vi "PID-control.vi"() -> ()   [LabVIEW 2012]
panel:
  out "Waveform Graph 2":dynamicdata(graph)
  in  "stop":bool
  out "Waveform Graph":dynamicdata(graph)
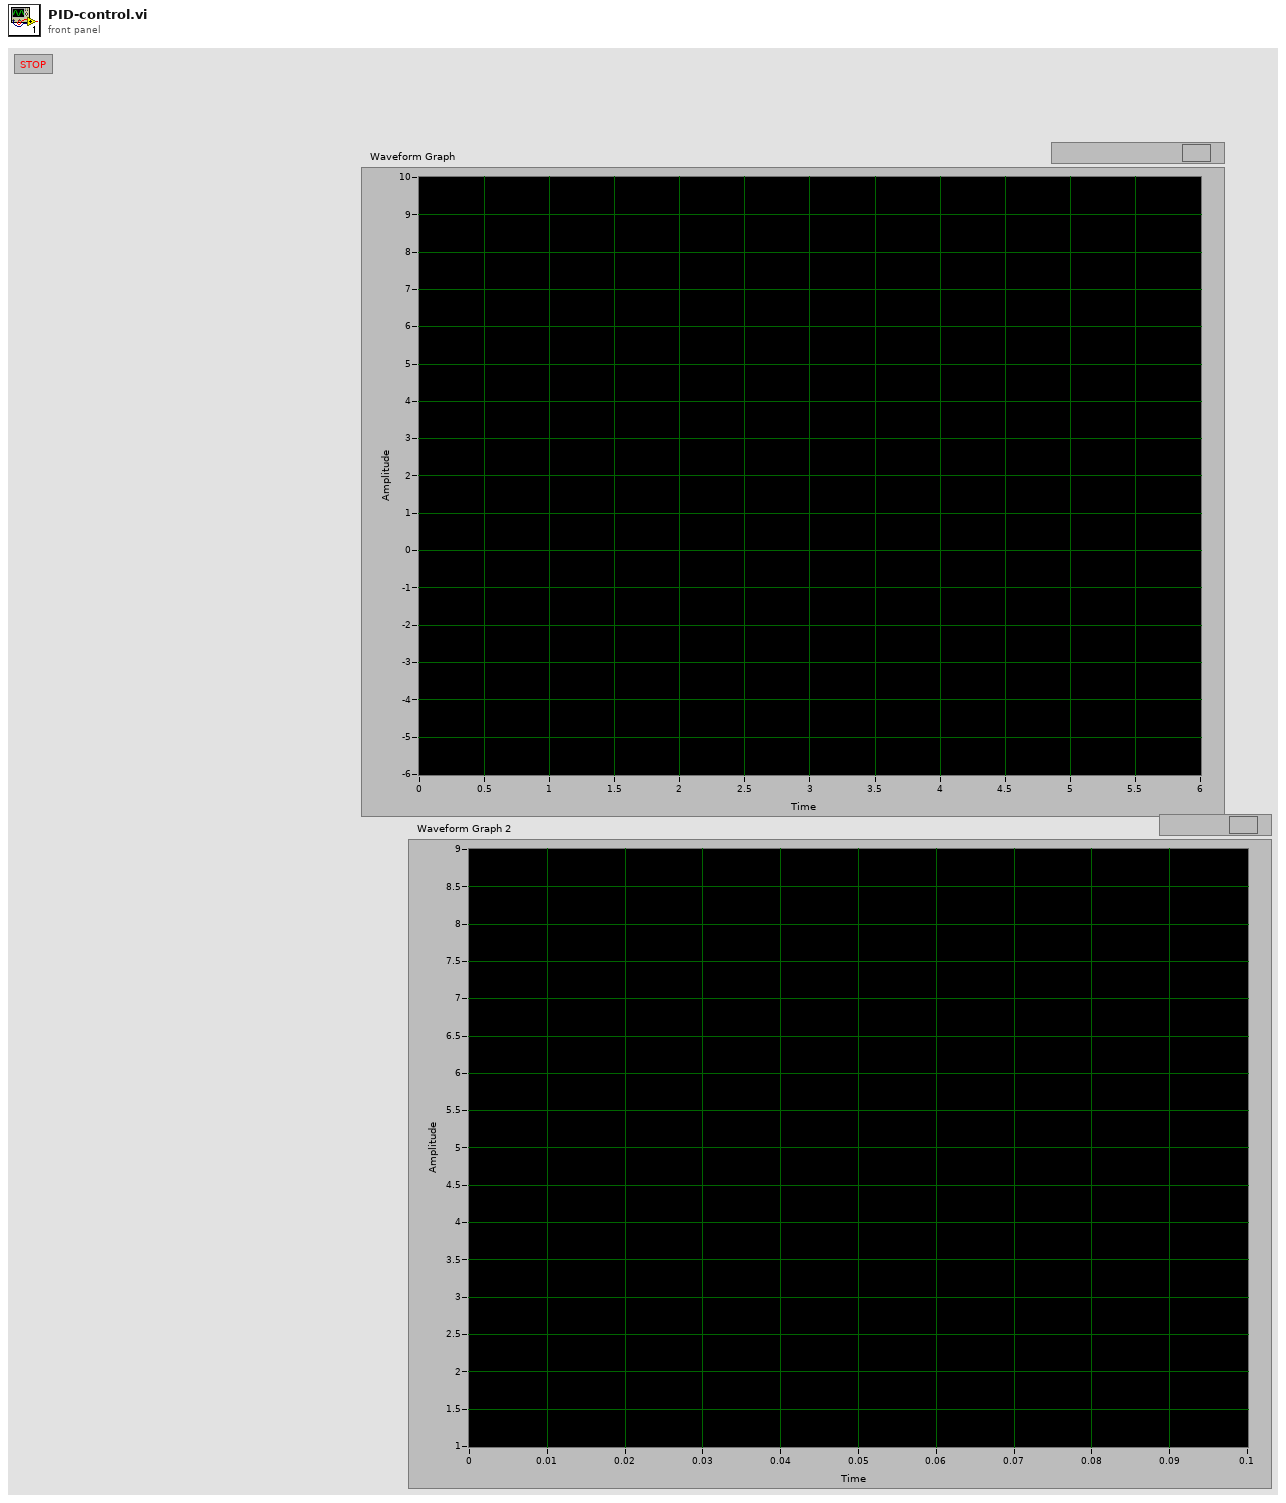
[diagram p1: front panel]
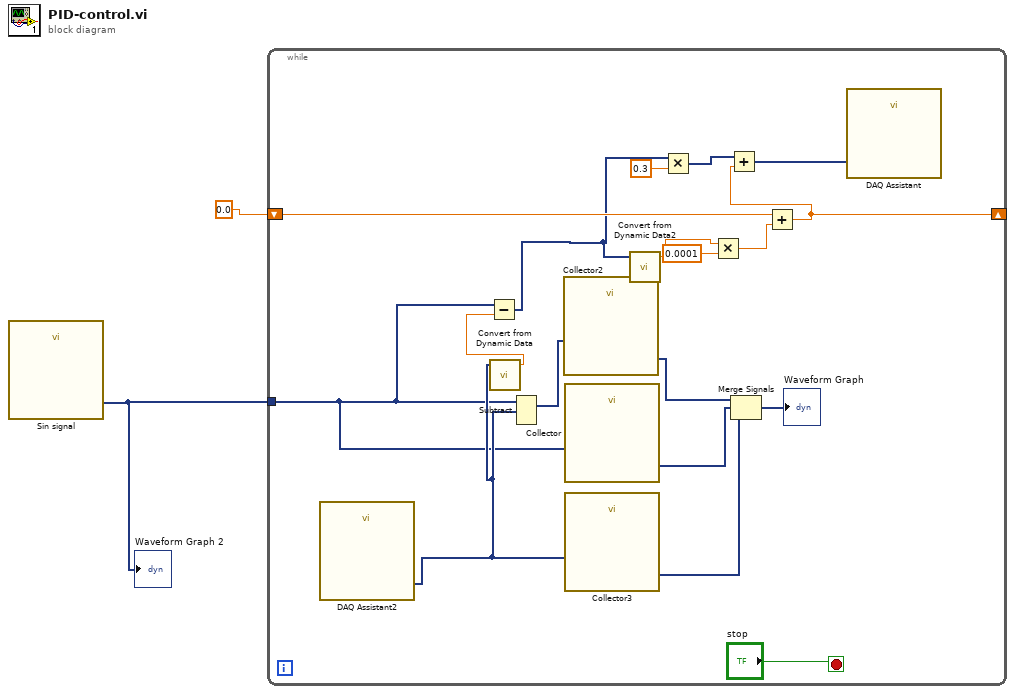
[diagram p0: block diagram]
diagram:
  n1 = call "Sin signal"() -> ("Triangle"=w2:dynamicdata)  [unwired: 14 in, 1 out]
  "Waveform Graph 2" <- w2
  n2 = while {
    shift-right: [w11] -> _
    shift-left: 0.0 ("y") -> [w15]
    tunnel: w2 -> [w6]
    stop <- "stop" stop-if-true
    n3 = call "DAQ Assistant2"() -> ("data"=w7:dynamicdata)  [unwired: 17 in, 2 out]
    n4 = call "Convert from Dynamic Data"("Dynamic Data Type"=w7) -> ("Scalar"=w5:dbl)  [unwired: 3 in]
    n5 = Subtract(x=w6, y=w5) -> (x-y=w4:dynamicdata)
    n6 = Subtract(1:w7, 2:w6) -> (0:w9:dynamicdata)  [unwired: 1 in, 1 out]
    n7 = call "Collector2"("Signals"=w9) -> ("Collected Signals"=w19:dynamicdata)  [unwired: 9 in, 1 out]
    n8 = call "Collector"("Signals"=w6) -> ("Collected Signals"=w17:dynamicdata)  [unwired: 9 in, 1 out]
    n9 = call "Collector3"("Signals"=w7) -> ("Collected Signals"=w16:dynamicdata)  [unwired: 9 in, 1 out]
    n10 = call "Convert from Dynamic Data2"("Dynamic Data Type"=w4) -> ("Scalar"=w3:dbl)  [unwired: 3 in]
    n11 = Multiply(x=w4, y=0.3) -> (x*y=w10:dynamicdata)
    n12 = Multiply(x=w3, y=0.0001) -> (x*y=w14:dbl)
    n13 = Merge Signals(w19, w17, w16) -> (→"Waveform Graph":dynamicdata)
    n14 = Add(x=w15, y=w14) -> (x+y=w11:dbl)
    n15 = Add(x=w10, y=w11) -> (x+y=w12:dynamicdata)
    n16 = call "DAQ Assistant"("data"=w12) -> ()  [unwired: 17 in, 2 out]
  }
